vi "メイン.vi"() -> (2 "測定周期/ms":dbl, 3 "値転記用配列":T2[](array[typedef]))   [LabVIEW 2021] (continued)
                      n5618 = global write "測定値MAXMIN_G.vi" "測定値MAX/MINグローバル"(w7929) -> ()
                    }
                  }
                }
                frame 5 {
                  n5619 = local read "測定新値\nリセット用 6"() -> (w7930:bool)
                  n5620 = local read "測定旧値 6"() -> (w7931:bool)
                  n5621 = case shown="TRUE" w7930 {
                    frame False {
                    }
                    frame True {
                      n5622 = property on="MAX/MINグローバルリセット用" class="Arr (指定)"() -> ("Value"=w7932:string[][])  [unwired: 2 in, 2 out]
                      n5623 = global write "測定値MAXMIN_G.vi" "測定値MAX/MINグローバル"(w7932) -> ()
                    }
                  }
                  n5624 = case shown="TRUE" w7931 {
                    frame False {
                    }
                    frame True {
                      n5625 = property on="MAX/MINグローバルリセット用" class="Arr (指定)"() -> ("Value"=w7933:string[][])  [unwired: 2 in, 2 out]
                      n5626 = global write "測定値MAXMIN_G.vi" "測定値MAX/MINグローバル"(w7933) -> ()
                    }
                  }
                }
                frame 7 {
                  n5627 = local read "測定新値\nリセット用 8"() -> (w7934:bool)
                  n5628 = local read "測定旧値 8"() -> (w7935:bool)
                  n5629 = case shown="TRUE" w7934 {
                    frame False {
                    }
                    frame True {
                      n5630 = property on="MAX/MINグローバルリセット用" class="Arr (指定)"() -> ("Value"=w7936:string[][])  [unwired: 2 in, 2 out]
                      n5631 = global write "測定値MAXMIN_G.vi" "測定値MAX/MINグローバル"(w7936) -> ()
                    }
                  }
                  n5632 = case shown="TRUE" w7935 {
                    frame False {
                    }
                    frame True {
                      n5633 = property on="MAX/MINグローバルリセット用" class="Arr (指定)"() -> ("Value"=w7937:string[][])  [unwired: 2 in, 2 out]
                      n5634 = global write "測定値MAXMIN_G.vi" "測定値MAX/MINグローバル"(w7937) -> ()
                    }
                  }
                }
                frame 8 {
                  n5635 = local read "測定新値\nリセット用 9"() -> (w7938:bool)
                  n5636 = local read "測定旧値 9"() -> (w7939:bool)
                  n5637 = case shown="TRUE" w7938 {
                    frame False {
                    }
                    frame True {
                      n5638 = property on="MAX/MINグローバルリセット用" class="Arr (指定)"() -> ("Value"=w7940:string[][])  [unwired: 2 in, 2 out]
                      n5639 = global write "測定値MAXMIN_G.vi" "測定値MAX/MINグローバル"(w7940) -> ()
                    }
                  }
                  n5640 = case shown="TRUE" w7939 {
                    frame False {
                    }
                    frame True {
                      n5641 = property on="MAX/MINグローバルリセット用" class="Arr (指定)"() -> ("Value"=w7941:string[][])  [unwired: 2 in, 2 out]
                      n5642 = global write "測定値MAXMIN_G.vi" "測定値MAX/MINグローバル"(w7941) -> ()
                    }
                  }
                }
                frame 9 {
                  n5643 = local read "測定新値\nリセット用 10"() -> (w7942:bool)
                  n5644 = local read "測定旧値 10"() -> (w7943:bool)
                  n5645 = case shown="TRUE" w7942 {
                    frame False {
                    }
                    frame True {
                      n5646 = property on="MAX/MINグローバルリセット用" class="Arr (指定)"() -> ("Value"=w7944:string[][])  [unwired: 2 in, 2 out]
                      n5647 = global write "測定値MAXMIN_G.vi" "測定値MAX/MINグローバル"(w7944) -> ()
                    }
                  }
                  n5648 = case shown="TRUE" w7943 {
                    frame False {
                    }
                    frame True {
                      n5649 = property on="MAX/MINグローバルリセット用" class="Arr (指定)"() -> ("Value"=w7945:string[][])  [unwired: 2 in, 2 out]
                      n5650 = global write "測定値MAXMIN_G.vi" "測定値MAX/MINグローバル"(w7945) -> ()
                    }
                  }
                }
                frame 10 {
                  n5651 = local read "測定新値\nリセット用 11"() -> (w7946:bool)
                  n5652 = local read "測定旧値 11"() -> (w7947:bool)
                  n5653 = case shown="TRUE" w7946 {
                    frame False {
                    }
                    frame True {
                      n5654 = property on="MAX/MINグローバルリセット用" class="Arr (指定)"() -> ("Value"=w7948:string[][])  [unwired: 2 in, 2 out]
                      n5655 = global write "測定値MAXMIN_G.vi" "測定値MAX/MINグローバル"(w7948) -> ()
                    }
                  }
                  n5656 = case shown="TRUE" w7947 {
                    frame False {
                    }
                    frame True {
                      n5657 = property on="MAX/MINグローバルリセット用" class="Arr (指定)"() -> ("Value"=w7949:string[][])  [unwired: 2 in, 2 out]
                      n5658 = global write "測定値MAXMIN_G.vi" "測定値MAX/MINグローバル"(w7949) -> ()
                    }
                  }
                }
                frame 11 {
                  n5659 = local read "測定新値\nリセット用 12"() -> (w7950:bool)
                  n5660 = local read "測定旧値 12"() -> (w7951:bool)
                  n5661 = case shown="TRUE" w7950 {
                    frame False {
                    }
                    frame True {
                      n5662 = property on="MAX/MINグローバルリセット用" class="Arr (指定)"() -> ("Value"=w7952:string[][])  [unwired: 2 in, 2 out]
                      n5663 = global write "測定値MAXMIN_G.vi" "測定値MAX/MINグローバル"(w7952) -> ()
                    }
                  }
                  n5664 = case shown="TRUE" w7951 {
                    frame False {
                    }
                    frame True {
                      n5665 = property on="MAX/MINグローバルリセット用" class="Arr (指定)"() -> ("Value"=w7953:string[][])  [unwired: 2 in, 2 out]
                      n5666 = global write "測定値MAXMIN_G.vi" "測定値MAX/MINグローバル"(w7953) -> ()
                    }
                  }
                }
              }
            }
          }
          frame #1 {
            w7954 = FALSE
            # "②測定新規リセット用、測定旧値のリセット"
            n5667 = global write "測定キャンセルボタン.vi" "グローバル_測定キャンセルボタン"(w7954) -> ()
            n5668 = local write "G_メイン測定キャンセルボタン"(w7954) -> ()
            n5669 = for {
              N: w7955 -> [_]
              tunnel: w7954 -> [w7959]
              i -> [w7960]
              n5670 = case shown="11" w7960 {
                tunnel: w7959 -> [w7961 w7962 w7963 w7964 w7965 w7966 w7967 w7968 w7969 w7970 w7971 w7972]
                frame 0, Default {
                  n5671 = local write "測定新値\nリセット用 1"(w7961) -> ()
                  n5672 = local write "測定旧値 1"(w7961) -> ()
                }
                frame 1 {
                  n5673 = local write "測定新値\nリセット用 2"(w7962) -> ()
                  n5674 = local write "測定旧値 2"(w7962) -> ()
                }
                frame 2 {
                  n5675 = local write "測定新値\nリセット用 3"(w7963) -> ()
                  n5676 = local write "測定旧値 3"(w7963) -> ()
                }
                frame 3 {
                  n5677 = local write "測定新値\nリセット用 4"(w7964) -> ()
                  n5678 = local write "測定旧値 4"(w7964) -> ()
                }
                frame 4 {
                  n5679 = local write "測定新値\nリセット用 5"(w7965) -> ()
                  n5680 = local write "測定旧値 5"(w7965) -> ()
                }
                frame 5 {
                  n5681 = local write "測定新値\nリセット用 6"(w7966) -> ()
                  n5682 = local write "測定旧値 6"(w7966) -> ()
                }
                frame 6 {
                  n5683 = local write "測定新値\nリセット用 7"(w7967) -> ()
                  n5684 = local write "測定旧値 7"(w7967) -> ()
                }
                frame 7 {
                  n5685 = local write "測定新値\nリセット用 8"(w7968) -> ()
                  n5686 = local write "測定旧値 8"(w7968) -> ()
                }
                frame 8 {
                  n5687 = local write "測定新値\nリセット用 9"(w7969) -> ()
                  n5688 = local write "測定旧値 9"(w7969) -> ()
                }
                frame 9 {
                  n5689 = local write "測定新値\nリセット用 10"(w7970) -> ()
                  n5690 = local write "測定旧値 10"(w7970) -> ()
                }
                frame 10 {
                  n5691 = local write "測定新値\nリセット用 11"(w7971) -> ()
                  n5692 = local write "測定旧値 11"(w7971) -> ()
                }
                frame 11 {
                  n5693 = local write "測定新値\nリセット用 12"(w7972) -> ()
                  n5694 = local write "測定旧値 12"(w7972) -> ()
                }
              }
            }
          }
          frame #2 {
            # "⑦キュー"
            # "④グローバル_測定キャンセルボタンを\n対象測定新値がFalseならTrueにする"
            n5695 = case shown="TRUE" w7975 {
              tunnel: [_ w7985] -> w7979
              tunnel: w7978 -> [_ w7984]
              tunnel: [_ w7983] -> w7977
              tunnel: w7976 -> [_ w7982]
              tunnel: [w7980 w7981] -> w7974
              tunnel: [w7980 w7981] -> w7973
              frame False {
                w7980 = TRUE
              }
              frame True {
                w7981 = TRUE
                n5696 = Enqueue Element(queue=w7984, element="測定7", error in (no error)=w7982) -> (queue out=w7985:refnum<queue>, error out=w7983:errorcluster)  [unwired: 1 in, 1 out]
              }
            }
            n5697 = local write "G_メイン測定キャンセルボタン"(w7974) -> ()
            n5698 = global write "測定キャンセルボタン.vi" "グローバル_測定キャンセルボタン"(w7973) -> ()
          }
        }
        n5699 = for {
          N: 12 -> [_]
          tunnel: w7877 -> [w7891]
          i -> [w7892]
          n5700 = case shown="11" w7892 {
            tunnel: w7891 -> [w7893 w7894 w7895 w7896 w7897 w7898 w7899 w7900 w7901 w7902 w7903 w7904]
            frame 0, Default {
              n5701 = property on="メイン測定ボタン_単発 1" class="Bool (指定)"("DisabledEnum"=w7893) -> ()  [unwired: 2 in, 2 out]
              n5702 = property on="メイン測定ボタン_連続 1" class="Bool (指定)"("DisabledEnum"=w7893) -> ()  [unwired: 2 in, 2 out]
            }
            frame 1 {
              n5703 = property on="メイン測定ボタン_単発 2" class="Bool (指定)"("DisabledEnum"=w7894) -> ()  [unwired: 2 in, 2 out]
              n5704 = property on="メイン測定ボタン_連続 2" class="Bool (指定)"("DisabledEnum"=w7894) -> ()  [unwired: 2 in, 2 out]
            }
            frame 2 {
              n5705 = property on="メイン測定ボタン_単発 3" class="Bool (指定)"("DisabledEnum"=w7895) -> ()  [unwired: 2 in, 2 out]
              n5706 = property on="メイン測定ボタン_連続 3" class="Bool (指定)"("DisabledEnum"=w7895) -> ()  [unwired: 2 in, 2 out]
            }
            frame 3 {
              n5707 = property on="メイン測定ボタン_単発 4" class="Bool (指定)"("DisabledEnum"=w7896) -> ()  [unwired: 2 in, 2 out]
              n5708 = property on="メイン測定ボタン_連続 4" class="Bool (指定)"("DisabledEnum"=w7896) -> ()  [unwired: 2 in, 2 out]
            }
            frame 4 {
              n5709 = property on="メイン測定ボタン_単発 5" class="Bool (指定)"("DisabledEnum"=w7897) -> ()  [unwired: 2 in, 2 out]
              n5710 = property on="メイン測定ボタン_連続 5" class="Bool (指定)"("DisabledEnum"=w7897) -> ()  [unwired: 2 in, 2 out]
            }
            frame 5 {
              n5711 = property on="メイン測定ボタン_連続 6" class="Bool (指定)"("DisabledEnum"=w7898) -> ()  [unwired: 2 in, 2 out]
              n5712 = property on="メイン測定ボタン_単発 6" class="Bool (指定)"("DisabledEnum"=w7898) -> ()  [unwired: 2 in, 2 out]
            }
            frame 6 {
              n5713 = property on="メイン測定ボタン_連続 7" class="Bool (指定)"("DisabledEnum"=w7899) -> ()  [unwired: 2 in, 2 out]
              n5714 = property on="メイン測定ボタン_単発 7" class="Bool (指定)"("DisabledEnum"=w7899) -> ()  [unwired: 2 in, 2 out]
            }
            frame 7 {
              n5715 = property on="メイン測定ボタン_単発 8" class="Bool (指定)"("DisabledEnum"=w7900) -> ()  [unwired: 2 in, 2 out]
              n5716 = property on="メイン測定ボタン_連続 8" class="Bool (指定)"("DisabledEnum"=w7900) -> ()  [unwired: 2 in, 2 out]
            }
            frame 8 {
              n5717 = property on="メイン測定ボタン_単発 9" class="Bool (指定)"("DisabledEnum"=w7901) -> ()  [unwired: 2 in, 2 out]
              n5718 = property on="メイン測定ボタン_連続 9" class="Bool (指定)"("DisabledEnum"=w7901) -> ()  [unwired: 2 in, 2 out]
            }
            frame 9 {
              n5719 = property on="メイン測定ボタン_単発 10" class="Bool (指定)"("DisabledEnum"=w7902) -> ()  [unwired: 2 in, 2 out]
              n5720 = property on="メイン測定ボタン_連続 10" class="Bool (指定)"("DisabledEnum"=w7902) -> ()  [unwired: 2 in, 2 out]
            }
            frame 10 {
              n5721 = property on="メイン測定ボタン_単発 11" class="Bool (指定)"("DisabledEnum"=w7903) -> ()  [unwired: 2 in, 2 out]
              n5722 = property on="メイン測定ボタン_連続 11" class="Bool (指定)"("DisabledEnum"=w7903) -> ()  [unwired: 2 in, 2 out]
            }
            frame 11 {
              n5723 = property on="メイン測定ボタン_連続 12" class="Bool (指定)"("DisabledEnum"=w7904) -> ()  [unwired: 2 in, 2 out]
              n5724 = property on="メイン測定ボタン_単発 12" class="Bool (指定)"("DisabledEnum"=w7904) -> ()  [unwired: 2 in, 2 out]
            }
          }
        }
        n5725 = property on="TOPページへ" class="Bool"("DisabledEnum"=w7877) -> ()  [unwired: 2 in, 2 out]
        n5726 = property on="保存して終了" class="Bool"("DisabledEnum"=w7877) -> ()  [unwired: 2 in, 2 out]
        n5727 = property on="保存せずに" class="Bool"("DisabledEnum"=w7877) -> ()  [unwired: 2 in, 2 out]
      }
      event Value Change {
        w7988 = T8."Disabled" ("無効")
        # "⑤"
        # "※複製時\n①このボタンで操作する以外の\n測定旧値\n測定新値\nを複製して作る\n②ある分だけの\n測定旧値\nを複製して作る\n③ある分だけの\n測定旧値\nを複製して作る\n④はそのまま\n⑤測定新値の\nボタンが複製されているか確認\n⑥Ⅰ.初期設定の\n測定新値_リセットの初期化\nを必ず作る事\n⑦キュー"
        # "単発測定ボタンを押した時、G_メインとグローバルのキャンセルボタンがFalseになり、連続測定が可能な状態になる。\n500ミリ秒後G_メインとグローバルのキャンセルボタンがTrueになり、連続測定が止まる"
        n5728 = event-data() -> ("NewVal"=w7997:T7)  [unwired: 1 in, 2 out]
        "測定新値 8" <- w7997
        n5729 = local read "書込周期/ms"() -> (w7987:dbl)
        n5730 = Wait (ms)(milliseconds to wait=w7987) -> ()  [unwired: 1 out]
        n5731 = flat-sequence {
          tunnel: w7997 -> [w8017]
          tunnel: w7998 -> [w8018]
          tunnel: w8000 -> [w8019]
          tunnel: [w8019] -> w7993
          tunnel: [w8018] -> w7992
          tunnel: [w8017] -> w7991
          tunnel: [w8016] -> w7990
          tunnel: [w8069] -> w7996
          tunnel: [w8068] -> w7995
          tunnel: [w8067] -> w7994
          tunnel: w7990 -> [w8066]
          tunnel: w7991 -> [w8067]
          tunnel: w7992 -> [w8068]
          tunnel: w7993 -> [w8069]
          tunnel: [w8090] -> w8001
          tunnel: [w8088] -> w7999
          tunnel: w7996 -> [w8089]
          tunnel: w7995 -> [w8087]
          tunnel: w7994 -> [w8086]
          frame #0 {
            w8016 = 32
            # "測定旧値・新値～32までTrueだったらMAX/MINグローバルリセット"
            # "①"
            n5732 = for {
              N: w8016 -> [_]
              i -> [w8020]
              n5733 = case shown="11" w8020 {
                frame 0, Default {
                  n5734 = local read "測定新値\nリセット用 1"() -> (w8021:bool)
                  n5735 = local read "測定旧値 1"() -> (w8022:bool)
                  n5736 = case shown="TRUE" w8021 {
                    frame False {
                    }
                    frame True {
                      n5737 = property on="MAX/MINグローバルリセット用" class="Arr (指定)"() -> ("Value"=w8023:string[][])  [unwired: 2 in, 2 out]
                      n5738 = global write "測定値MAXMIN_G.vi" "測定値MAX/MINグローバル"(w8023) -> ()
                    }
                  }
                  n5739 = case shown="TRUE" w8022 {
                    frame False {
                    }
                    frame True {
                      n5740 = property on="MAX/MINグローバルリセット用" class="Arr (指定)"() -> ("Value"=w8024:string[][])  [unwired: 2 in, 2 out]
                      n5741 = global write "測定値MAXMIN_G.vi" "測定値MAX/MINグローバル"(w8024) -> ()
                    }
                  }
                }
                frame 1 {
                  n5742 = local read "測定新値\nリセット用 2"() -> (w8025:bool)
                  n5743 = local read "測定旧値 2"() -> (w8026:bool)
                  n5744 = case shown="TRUE" w8025 {
                    frame False {
                    }
                    frame True {
                      n5745 = property on="MAX/MINグローバルリセット用" class="Arr (指定)"() -> ("Value"=w8027:string[][])  [unwired: 2 in, 2 out]
                      n5746 = global write "測定値MAXMIN_G.vi" "測定値MAX/MINグローバル"(w8027) -> ()
                    }
                  }
                  n5747 = case shown="TRUE" w8026 {
                    frame False {
                    }
                    frame True {
                      n5748 = property on="MAX/MINグローバルリセット用" class="Arr (指定)"() -> ("Value"=w8028:string[][])  [unwired: 2 in, 2 out]
                      n5749 = global write "測定値MAXMIN_G.vi" "測定値MAX/MINグローバル"(w8028) -> ()
                    }
                  }
                }
                frame 2 {
                  n5750 = local read "測定新値\nリセット用 3"() -> (w8029:bool)
                  n5751 = local read "測定旧値 3"() -> (w8030:bool)
                  n5752 = case shown="TRUE" w8029 {
                    frame False {
                    }
                    frame True {
                      n5753 = property on="MAX/MINグローバルリセット用" class="Arr (指定)"() -> ("Value"=w8031:string[][])  [unwired: 2 in, 2 out]
                      n5754 = global write "測定値MAXMIN_G.vi" "測定値MAX/MINグローバル"(w8031) -> ()
                    }
                  }
                  n5755 = case shown="TRUE" w8030 {
                    frame False {
                    }
                    frame True {
                      n5756 = property on="MAX/MINグローバルリセット用" class="Arr (指定)"() -> ("Value"=w8032:string[][])  [unwired: 2 in, 2 out]
                      n5757 = global write "測定値MAXMIN_G.vi" "測定値MAX/MINグローバル"(w8032) -> ()
                    }
                  }
                }
                frame 3 {
                  n5758 = local read "測定新値\nリセット用 4"() -> (w8033:bool)
                  n5759 = local read "測定旧値 4"() -> (w8034:bool)
                  n5760 = case shown="TRUE" w8033 {
                    frame False {
                    }
                    frame True {
                      n5761 = property on="MAX/MINグローバルリセット用" class="Arr (指定)"() -> ("Value"=w8035:string[][])  [unwired: 2 in, 2 out]
                      n5762 = global write "測定値MAXMIN_G.vi" "測定値MAX/MINグローバル"(w8035) -> ()
                    }
                  }
                  n5763 = case shown="TRUE" w8034 {
                    frame False {
                    }
                    frame True {
                      n5764 = property on="MAX/MINグローバルリセット用" class="Arr (指定)"() -> ("Value"=w8036:string[][])  [unwired: 2 in, 2 out]
                      n5765 = global write "測定値MAXMIN_G.vi" "測定値MAX/MINグローバル"(w8036) -> ()
                    }
                  }
                }
                frame 4 {
                  n5766 = local read "測定新値\nリセット用 5"() -> (w8037:bool)
                  n5767 = local read "測定旧値 5"() -> (w8038:bool)
                  n5768 = case shown="TRUE" w8037 {
                    frame False {
                    }
                    frame True {
                      n5769 = property on="MAX/MINグローバルリセット用" class="Arr (指定)"() -> ("Value"=w8039:string[][])  [unwired: 2 in, 2 out]
                      n5770 = global write "測定値MAXMIN_G.vi" "測定値MAX/MINグローバル"(w8039) -> ()
                    }
                  }
                  n5771 = case shown="TRUE" w8038 {
                    frame False {
                    }
                    frame True {
                      n5772 = property on="MAX/MINグローバルリセット用" class="Arr (指定)"() -> ("Value"=w8040:string[][])  [unwired: 2 in, 2 out]
                      n5773 = global write "測定値MAXMIN_G.vi" "測定値MAX/MINグローバル"(w8040) -> ()
                    }
                  }
                }
                frame 5 {
                  n5774 = local read "測定新値\nリセット用 6"() -> (w8041:bool)
                  n5775 = local read "測定旧値 6"() -> (w8042:bool)
                  n5776 = case shown="TRUE" w8041 {
                    frame False {
                    }
                    frame True {
                      n5777 = property on="MAX/MINグローバルリセット用" class="Arr (指定)"() -> ("Value"=w8043:string[][])  [unwired: 2 in, 2 out]
                      n5778 = global write "測定値MAXMIN_G.vi" "測定値MAX/MINグローバル"(w8043) -> ()
                    }
                  }
                  n5779 = case shown="TRUE" w8042 {
                    frame False {
                    }
                    frame True {
                      n5780 = property on="MAX/MINグローバルリセット用" class="Arr (指定)"() -> ("Value"=w8044:string[][])  [unwired: 2 in, 2 out]
                      n5781 = global write "測定値MAXMIN_G.vi" "測定値MAX/MINグローバル"(w8044) -> ()
                    }
                  }
                }
                frame 6 {
                  n5782 = local read "測定新値\nリセット用 7"() -> (w8045:bool)
                  n5783 = local read "測定旧値 7"() -> (w8046:bool)
                  n5784 = case shown="TRUE" w8045 {
                    frame False {
                    }
                    frame True {
                      n5785 = property on="MAX/MINグローバルリセット用" class="Arr (指定)"() -> ("Value"=w8047:string[][])  [unwired: 2 in, 2 out]
                      n5786 = global write "測定値MAXMIN_G.vi" "測定値MAX/MINグローバル"(w8047) -> ()
                    }
                  }
                  n5787 = case shown="TRUE" w8046 {
                    frame False {
                    }
                    frame True {
                      n5788 = property on="MAX/MINグローバルリセット用" class="Arr (指定)"() -> ("Value"=w8048:string[][])  [unwired: 2 in, 2 out]
                      n5789 = global write "測定値MAXMIN_G.vi" "測定値MAX/MINグローバル"(w8048) -> ()
                    }
                  }
                }
                frame 8 {
                  n5790 = local read "測定新値\nリセット用 9"() -> (w8049:bool)
                  n5791 = local read "測定旧値 9"() -> (w8050:bool)
                  n5792 = case shown="TRUE" w8049 {
                    frame False {
                    }
                    frame True {
                      n5793 = property on="MAX/MINグローバルリセット用" class="Arr (指定)"() -> ("Value"=w8051:string[][])  [unwired: 2 in, 2 out]
                      n5794 = global write "測定値MAXMIN_G.vi" "測定値MAX/MINグローバル"(w8051) -> ()
                    }
                  }
                  n5795 = case shown="TRUE" w8050 {
                    frame False {
                    }
                    frame True {
                      n5796 = property on="MAX/MINグローバルリセット用" class="Arr (指定)"() -> ("Value"=w8052:string[][])  [unwired: 2 in, 2 out]
                      n5797 = global write "測定値MAXMIN_G.vi" "測定値MAX/MINグローバル"(w8052) -> ()
                    }
                  }
                }
                frame 9 {
                  n5798 = local read "測定新値\nリセット用 10"() -> (w8053:bool)
                  n5799 = local read "測定旧値 10"() -> (w8054:bool)
                  n5800 = case shown="TRUE" w8053 {
                    frame False {
                    }
                    frame True {
                      n5801 = property on="MAX/MINグローバルリセット用" class="Arr (指定)"() -> ("Value"=w8055:string[][])  [unwired: 2 in, 2 out]
                      n5802 = global write "測定値MAXMIN_G.vi" "測定値MAX/MINグローバル"(w8055) -> ()
                    }
                  }
                  n5803 = case shown="TRUE" w8054 {
                    frame False {
                    }
                    frame True {
                      n5804 = property on="MAX/MINグローバルリセット用" class="Arr (指定)"() -> ("Value"=w8056:string[][])  [unwired: 2 in, 2 out]
                      n5805 = global write "測定値MAXMIN_G.vi" "測定値MAX/MINグローバル"(w8056) -> ()
                    }
                  }
                }
                frame 10 {
                  n5806 = local read "測定新値\nリセット用 11"() -> (w8057:bool)
                  n5807 = local read "測定旧値 11"() -> (w8058:bool)
                  n5808 = case shown="TRUE" w8057 {
                    frame False {
                    }
                    frame True {
                      n5809 = property on="MAX/MINグローバルリセット用" class="Arr (指定)"() -> ("Value"=w8059:string[][])  [unwired: 2 in, 2 out]
                      n5810 = global write "測定値MAXMIN_G.vi" "測定値MAX/MINグローバル"(w8059) -> ()
                    }
                  }
                  n5811 = case shown="TRUE" w8058 {
                    frame False {
                    }
                    frame True {
                      n5812 = property on="MAX/MINグローバルリセット用" class="Arr (指定)"() -> ("Value"=w8060:string[][])  [unwired: 2 in, 2 out]
                      n5813 = global write "測定値MAXMIN_G.vi" "測定値MAX/MINグローバル"(w8060) -> ()
                    }
                  }
                }
                frame 11 {
                  n5814 = local read "測定新値\nリセット用 12"() -> (w8061:bool)
                  n5815 = local read "測定旧値 12"() -> (w8062:bool)
                  n5816 = case shown="TRUE" w8061 {
                    frame False {
                    }
                    frame True {
                      n5817 = property on="MAX/MINグローバルリセット用" class="Arr (指定)"() -> ("Value"=w8063:string[][])  [unwired: 2 in, 2 out]
                      n5818 = global write "測定値MAXMIN_G.vi" "測定値MAX/MINグローバル"(w8063) -> ()
                    }
                  }
                  n5819 = case shown="TRUE" w8062 {
                    frame False {
                    }
                    frame True {
                      n5820 = property on="MAX/MINグローバルリセット用" class="Arr (指定)"() -> ("Value"=w8064:string[][])  [unwired: 2 in, 2 out]
                      n5821 = global write "測定値MAXMIN_G.vi" "測定値MAX/MINグローバル"(w8064) -> ()
                    }
                  }
                }
              }
            }
          }
          frame #1 {
            w8065 = FALSE
            # "②測定新規リセット用、測定旧値のリセット"
            n5822 = global write "測定キャンセルボタン.vi" "グローバル_測定キャンセルボタン"(w8065) -> ()
            n5823 = local write "G_メイン測定キャンセルボタン"(w8065) -> ()
            n5824 = for {
              N: w8066 -> [_]
              tunnel: w8065 -> [w8070]
              i -> [w8071]
              n5825 = case shown="11" w8071 {
                tunnel: w8070 -> [w8072 w8073 w8074 w8075 w8076 w8077 w8078 w8079 w8080 w8081 w8082 w8083]
                frame 0, Default {
                  n5826 = local write "測定新値\nリセット用 1"(w8072) -> ()
                  n5827 = local write "測定旧値 1"(w8072) -> ()
                }
                frame 1 {
                  n5828 = local write "測定新値\nリセット用 2"(w8073) -> ()
                  n5829 = local write "測定旧値 2"(w8073) -> ()
                }
                frame 2 {
                  n5830 = local write "測定新値\nリセット用 3"(w8074) -> ()
                  n5831 = local write "測定旧値 3"(w8074) -> ()
                }
                frame 3 {
                  n5832 = local write "測定新値\nリセット用 4"(w8075) -> ()
                  n5833 = local write "測定旧値 4"(w8075) -> ()
                }
                frame 4 {
                  n5834 = local write "測定新値\nリセット用 5"(w8076) -> ()
                  n5835 = local write "測定旧値 5"(w8076) -> ()
                }
                frame 5 {
                  n5836 = local write "測定新値\nリセット用 6"(w8077) -> ()
                  n5837 = local write "測定旧値 6"(w8077) -> ()
                }
                frame 6 {
                  n5838 = local write "測定新値\nリセット用 7"(w8078) -> ()
                  n5839 = local write "測定旧値 7"(w8078) -> ()
                }
                frame 7 {
                  n5840 = local write "測定新値\nリセット用 8"(w8079) -> ()
                  n5841 = local write "測定旧値 8"(w8079) -> ()
                }
                frame 8 {
                  n5842 = local write "測定新値\nリセット用 9"(w8080) -> ()
                  n5843 = local write "測定旧値 9"(w8080) -> ()
                }
                frame 9 {
                  n5844 = local write "測定新値\nリセット用 10"(w8081) -> ()
                  n5845 = local write "測定旧値 10"(w8081) -> ()
                }
                frame 10 {
                  n5846 = local write "測定新値\nリセット用 11"(w8082) -> ()
                  n5847 = local write "測定旧値 11"(w8082) -> ()
                }
                frame 11 {
                  n5848 = local write "測定新値\nリセット用 12"(w8083) -> ()
                  n5849 = local write "測定旧値 12"(w8083) -> ()
                }
              }
            }
          }
          frame #2 {
            # "⑦キュー"
            # "④グローバル_測定キャンセルボタンを\n対象測定新値がFalseならTrueにする"
            n5850 = case shown="TRUE" w8086 {
              tunnel: [_ w8096] -> w8090
              tunnel: w8089 -> [_ w8095]
              tunnel: [_ w8094] -> w8088
              tunnel: w8087 -> [_ w8093]
              tunnel: [w8091 w8092] -> w8085
              tunnel: [w8091 w8092] -> w8084
              frame False {
                w8091 = TRUE
              }
              frame True {
                w8092 = TRUE
                n5851 = Enqueue Element(queue=w8095, element="測定8", error in (no error)=w8093) -> (queue out=w8096:refnum<queue>, error out=w8094:errorcluster)  [unwired: 1 in, 1 out]
              }
            }
            n5852 = local write "G_メイン測定キャンセルボタン"(w8085) -> ()
            n5853 = global write "測定キャンセルボタン.vi" "グローバル_測定キャンセルボタン"(w8084) -> ()
          }
        }
        n5854 = for {
          N: 12 -> [_]
          tunnel: w7988 -> [w8002]
          i -> [w8003]
          n5855 = case shown="11" w8003 {
            tunnel: w8002 -> [w8004 w8005 w8006 w8007 w8008 w8009 w8010 w8011 w8012 w8013 w8014 w8015]
            frame 0, Default {
              n5856 = property on="メイン測定ボタン_単発 1" class="Bool (指定)"("DisabledEnum"=w8004) -> ()  [unwired: 2 in, 2 out]
              n5857 = property on="メイン測定ボタン_連続 1" class="Bool (指定)"("DisabledEnum"=w8004) -> ()  [unwired: 2 in, 2 out]
            }
            frame 1 {
              n5858 = property on="メイン測定ボタン_単発 2" class="Bool (指定)"("DisabledEnum"=w8005) -> ()  [unwired: 2 in, 2 out]
              n5859 = property on="メイン測定ボタン_連続 2" class="Bool (指定)"("DisabledEnum"=w8005) -> ()  [unwired: 2 in, 2 out]
            }
            frame 2 {
              n5860 = property on="メイン測定ボタン_単発 3" class="Bool (指定)"("DisabledEnum"=w8006) -> ()  [unwired: 2 in, 2 out]
              n5861 = property on="メイン測定ボタン_連続 3" class="Bool (指定)"("DisabledEnum"=w8006) -> ()  [unwired: 2 in, 2 out]
            }
            frame 3 {
              n5862 = property on="メイン測定ボタン_単発 4" class="Bool (指定)"("DisabledEnum"=w8007) -> ()  [unwired: 2 in, 2 out]
              n5863 = property on="メイン測定ボタン_連続 4" class="Bool (指定)"("DisabledEnum"=w8007) -> ()  [unwired: 2 in, 2 out]
            }
            frame 4 {
              n5864 = property on="メイン測定ボタン_単発 5" class="Bool (指定)"("DisabledEnum"=w8008) -> ()  [unwired: 2 in, 2 out]
              n5865 = property on="メイン測定ボタン_連続 5" class="Bool (指定)"("DisabledEnum"=w8008) -> ()  [unwired: 2 in, 2 out]
            }
            frame 5 {
              n5866 = property on="メイン測定ボタン_連続 6" class="Bool (指定)"("DisabledEnum"=w8009) -> ()  [unwired: 2 in, 2 out]
              n5867 = property on="メイン測定ボタン_単発 6" class="Bool (指定)"("DisabledEnum"=w8009) -> ()  [unwired: 2 in, 2 out]
            }
            frame 6 {
              n5868 = property on="メイン測定ボタン_連続 7" class="Bool (指定)"("DisabledEnum"=w8010) -> ()  [unwired: 2 in, 2 out]
              n5869 = property on="メイン測定ボタン_単発 7" class="Bool (指定)"("DisabledEnum"=w8010) -> ()  [unwired: 2 in, 2 out]
            }
            frame 7 {
              n5870 = property on="メイン測定ボタン_単発 8" class="Bool (指定)"("DisabledEnum"=w8011) -> ()  [unwired: 2 in, 2 out]
              n5871 = property on="メイン測定ボタン_連続 8" class="Bool (指定)"("DisabledEnum"=w8011) -> ()  [unwired: 2 in, 2 out]
            }
            frame 8 {
              n5872 = property on="メイン測定ボタン_単発 9" class="Bool (指定)"("DisabledEnum"=w8012) -> ()  [unwired: 2 in, 2 out]
              n5873 = property on="メイン測定ボタン_連続 9" class="Bool (指定)"("DisabledEnum"=w8012) -> ()  [unwired: 2 in, 2 out]
            }
            frame 9 {
              n5874 = property on="メイン測定ボタン_単発 10" class="Bool (指定)"("DisabledEnum"=w8013) -> ()  [unwired: 2 in, 2 out]
              n5875 = property on="メイン測定ボタン_連続 10" class="Bool (指定)"("DisabledEnum"=w8013) -> ()  [unwired: 2 in, 2 out]
            }
            frame 10 {
              n5876 = property on="メイン測定ボタン_単発 11" class="Bool (指定)"("DisabledEnum"=w8014) -> ()  [unwired: 2 in, 2 out]
              n5877 = property on="メイン測定ボタン_連続 11" class="Bool (指定)"("DisabledEnum"=w8014) -> ()  [unwired: 2 in, 2 out]
            }
            frame 11 {
              n5878 = property on="メイン測定ボタン_連続 12" class="Bool (指定)"("DisabledEnum"=w8015) -> ()  [unwired: 2 in, 2 out]
              n5879 = property on="メイン測定ボタン_単発 12" class="Bool (指定)"("DisabledEnum"=w8015) -> ()  [unwired: 2 in, 2 out]
            }
          }
        }
        n5880 = property on="TOPページへ" class="Bool"("DisabledEnum"=w7988) -> ()  [unwired: 2 in, 2 out]
        n5881 = property on="保存して終了" class="Bool"("DisabledEnum"=w7988) -> ()  [unwired: 2 in, 2 out]
        n5882 = property on="保存せずに" class="Bool"("DisabledEnum"=w7988) -> ()  [unwired: 2 in, 2 out]
      }
      event Value Change {
        w8099 = T8."Disabled" ("無効")
        # "⑤"
        # "※複製時\n①このボタンで操作する以外の\n測定旧値\n測定新値\nを複製して作る\n②ある分だけの\n測定旧値\nを複製して作る\n③ある分だけの\n測定旧値\nを複製して作る\n④はそのまま\n⑤測定新値の\nボタンが複製されているか確認\n⑥Ⅰ.初期設定の\n測定新値_リセットの初期化\nを必ず作る事\n⑦キュー\n⑧ループカウント"
        # "単発測定ボタンを押した時、G_メインとグローバルのキャンセルボタンがFalseになり、連続測定が可能な状態になる。\n500ミリ秒後G_メインとグローバルのキャンセルボタンがTrueになり、連続測定が止まる"
        n5883 = event-data() -> ("NewVal"=w8108:T7)  [unwired: 1 in, 2 out]
        "測定新値 9" <- w8108
        n5884 = local read "書込周期/ms"() -> (w8098:dbl)
        n5885 = Wait (ms)(milliseconds to wait=w8098) -> ()  [unwired: 1 out]
        n5886 = flat-sequence {
          tunnel: w8108 -> [w8128]
          tunnel: w8109 -> [w8129]
          tunnel: w8111 -> [w8130]
          tunnel: [w8130] -> w8104
          tunnel: [w8129] -> w8103
          tunnel: [w8128] -> w8102
          tunnel: [w8127] -> w8101
          tunnel: [w8180] -> w8107
          tunnel: [w8179] -> w8106
          tunnel: [w8178] -> w8105
          tunnel: w8101 -> [w8177]
          tunnel: w8102 -> [w8178]
          tunnel: w8103 -> [w8179]
          tunnel: w8104 -> [w8180]
          tunnel: [w8201] -> w8112
          tunnel: [w8199] -> w8110
          tunnel: w8107 -> [w8200]
          tunnel: w8106 -> [w8198]
          tunnel: w8105 -> [w8197]
          frame #0 {
            w8127 = 32
            # "⑧"
            # "測定旧値・新値～32までTrueだったらMAX/MINグローバルリセット"
            # "①"
            n5887 = for {
              N: w8127 -> [_]
              i -> [w8131]
              n5888 = case shown="11" w8131 {
                frame 0, Default {
                  n5889 = local read "測定新値\nリセット用 1"() -> (w8132:bool)
                  n5890 = local read "測定旧値 1"() -> (w8133:bool)
                  n5891 = case shown="FALSE" w8132 {
                    frame False {
                    }
                    frame True {
                      n5892 = property on="MAX/MINグローバルリセット用" class="Arr (指定)"() -> ("Value"=w8134:string[][])  [unwired: 2 in, 2 out]
                      n5893 = global write "測定値MAXMIN_G.vi" "測定値MAX/MINグローバル"(w8134) -> ()
                    }
                  }
                  n5894 = case shown="FALSE" w8133 {
                    frame False {
                    }
                    frame True {
                      n5895 = property on="MAX/MINグローバルリセット用" class="Arr (指定)"() -> ("Value"=w8135:string[][])  [unwired: 2 in, 2 out]
                      n5896 = global write "測定値MAXMIN_G.vi" "測定値MAX/MINグローバル"(w8135) -> ()
                    }
                  }
                }
                frame 1 {
                  n5897 = local read "測定新値\nリセット用 2"() -> (w8136:bool)
                  n5898 = local read "測定旧値 2"() -> (w8137:bool)
                  n5899 = case shown="FALSE" w8136 {
                    frame False {
                    }
                    frame True {
                      n5900 = property on="MAX/MINグローバルリセット用" class="Arr (指定)"() -> ("Value"=w8138:string[][])  [unwired: 2 in, 2 out]
                      n5901 = global write "測定値MAXMIN_G.vi" "測定値MAX/MINグローバル"(w8138) -> ()
                    }
                  }
                  n5902 = case shown="FALSE" w8137 {
                    frame False {
                    }
                    frame True {
                      n5903 = property on="MAX/MINグローバルリセット用" class="Arr (指定)"() -> ("Value"=w8139:string[][])  [unwired: 2 in, 2 out]
                      n5904 = global write "測定値MAXMIN_G.vi" "測定値MAX/MINグローバル"(w8139) -> ()
                    }
                  }
                }
                frame 2 {
                  n5905 = local read "測定新値\nリセット用 3"() -> (w8140:bool)
                  n5906 = local read "測定旧値 3"() -> (w8141:bool)
                  n5907 = case shown="FALSE" w8140 {
                    frame False {
                    }
                    frame True {
                      n5908 = property on="MAX/MINグローバルリセット用" class="Arr (指定)"() -> ("Value"=w8142:string[][])  [unwired: 2 in, 2 out]
                      n5909 = global write "測定値MAXMIN_G.vi" "測定値MAX/MINグローバル"(w8142) -> ()
                    }
                  }
                  n5910 = case shown="FALSE" w8141 {
                    frame False {
                    }
                    frame True {
                      n5911 = property on="MAX/MINグローバルリセット用" class="Arr (指定)"() -> ("Value"=w8143:string[][])  [unwired: 2 in, 2 out]
                      n5912 = global write "測定値MAXMIN_G.vi" "測定値MAX/MINグローバル"(w8143) -> ()
                    }
                  }
                }
                frame 3 {
                  n5913 = local read "測定新値\nリセット用 4"() -> (w8144:bool)
                  n5914 = local read "測定旧値 4"() -> (w8145:bool)
                  n5915 = case shown="FALSE" w8144 {
                    frame False {
                    }
                    frame True {
                      n5916 = property on="MAX/MINグローバルリセット用" class="Arr (指定)"() -> ("Value"=w8146:string[][])  [unwired: 2 in, 2 out]
                      n5917 = global write "測定値MAXMIN_G.vi" "測定値MAX/MINグローバル"(w8146) -> ()
                    }
                  }
                  n5918 = case shown="FALSE" w8145 {
                    frame False {
                    }
                    frame True {
                      n5919 = property on="MAX/MINグローバルリセット用" class="Arr (指定)"() -> ("Value"=w8147:string[][])  [unwired: 2 in, 2 out]
                      n5920 = global write "測定値MAXMIN_G.vi" "測定値MAX/MINグローバル"(w8147) -> ()
                    }
                  }
                }
                frame 4 {
                  n5921 = local read "測定新値\nリセット用 5"() -> (w8148:bool)
                  n5922 = local read "測定旧値 5"() -> (w8149:bool)
                  n5923 = case shown="FALSE" w8148 {
                    frame False {
                    }
                    frame True {
                      n5924 = property on="MAX/MINグローバルリセット用" class="Arr (指定)"() -> ("Value"=w8150:string[][])  [unwired: 2 in, 2 out]
                      n5925 = global write "測定値MAXMIN_G.vi" "測定値MAX/MINグローバル"(w8150) -> ()
                    }
                  }
                  n5926 = case shown="FALSE" w8149 {
                    frame False {
                    }
                    frame True {
                      n5927 = property on="MAX/MINグローバルリセット用" class="Arr (指定)"() -> ("Value"=w8151:string[][])  [unwired: 2 in, 2 out]
                      n5928 = global write "測定値MAXMIN_G.vi" "測定値MAX/MINグローバル"(w8151) -> ()
                    }
                  }
                }
                frame 5 {
                  n5929 = local read "測定新値\nリセット用 6"() -> (w8152:bool)
                  n5930 = local read "測定旧値 6"() -> (w8153:bool)
                  n5931 = case shown="FALSE" w8152 {
                    frame False {
                    }
                    frame True {
                      n5932 = property on="MAX/MINグローバルリセット用" class="Arr (指定)"() -> ("Value"=w8154:string[][])  [unwired: 2 in, 2 out]
                      n5933 = global write "測定値MAXMIN_G.vi" "測定値MAX/MINグローバル"(w8154) -> ()
                    }
                  }
                  n5934 = case shown="FALSE" w8153 {
                    frame False {
                    }
                    frame True {
                      n5935 = property on="MAX/MINグローバルリセット用" class="Arr (指定)"() -> ("Value"=w8155:string[][])  [unwired: 2 in, 2 out]
                      n5936 = global write "測定値MAXMIN_G.vi" "測定値MAX/MINグローバル"(w8155) -> ()
                    }
                  }
                }
                frame 6 {
                  n5937 = local read "測定新値\nリセット用 7"() -> (w8156:bool)
                  n5938 = local read "測定旧値 7"() -> (w8157:bool)
                  n5939 = case shown="FALSE" w8156 {
                    frame False {
                    }
                    frame True {
                      n5940 = property on="MAX/MINグローバルリセット用" class="Arr (指定)"() -> ("Value"=w8158:string[][])  [unwired: 2 in, 2 out]
                      n5941 = global write "測定値MAXMIN_G.vi" "測定値MAX/MINグローバル"(w8158) -> ()
                    }
                  }
                  n5942 = case shown="FALSE" w8157 {
                    frame False {
                    }
                    frame True {
                      n5943 = property on="MAX/MINグローバルリセット用" class="Arr (指定)"() -> ("Value"=w8159:string[][])  [unwired: 2 in, 2 out]
                      n5944 = global write "測定値MAXMIN_G.vi" "測定値MAX/MINグローバル"(w8159) -> ()
                    }
                  }
                }
                frame 7 {
                  n5945 = local read "測定新値\nリセット用 8"() -> (w8160:bool)
                  n5946 = local read "測定旧値 8"() -> (w8161:bool)
                  n5947 = case shown="TRUE" w8160 {
                    frame False {
                    }
                    frame True {
                      n5948 = property on="MAX/MINグローバルリセット用" class="Arr (指定)"() -> ("Value"=w8162:string[][])  [unwired: 2 in, 2 out]
                      n5949 = global write "測定値MAXMIN_G.vi" "測定値MAX/MINグローバル"(w8162) -> ()
                    }
                  }
                  n5950 = case shown="TRUE" w8161 {
                    frame False {
                    }
                    frame True {
                      n5951 = property on="MAX/MINグローバルリセット用" class="Arr (指定)"() -> ("Value"=w8163:string[][])  [unwired: 2 in, 2 out]
                      n5952 = global write "測定値MAXMIN_G.vi" "測定値MAX/MINグローバル"(w8163) -> ()
                    }
                  }
                }
                frame 9 {
                  n5953 = local read "測定新値\nリセット用 10"() -> (w8164:bool)
                  n5954 = local read "測定旧値 10"() -> (w8165:bool)
                  n5955 = case shown="TRUE" w8164 {
                    frame False {
                    }
                    frame True {
                      n5956 = property on="MAX/MINグローバルリセット用" class="Arr (指定)"() -> ("Value"=w8166:string[][])  [unwired: 2 in, 2 out]
                      n5957 = global write "測定値MAXMIN_G.vi" "測定値MAX/MINグローバル"(w8166) -> ()
                    }
                  }
                  n5958 = case shown="TRUE" w8165 {
                    frame False {
                    }
                    frame True {
                      n5959 = property on="MAX/MINグローバルリセット用" class="Arr (指定)"() -> ("Value"=w8167:string[][])  [unwired: 2 in, 2 out]
                      n5960 = global write "測定値MAXMIN_G.vi" "測定値MAX/MINグローバル"(w8167) -> ()
                    }
                  }
                }
                frame 10 {
                  n5961 = local read "測定新値\nリセット用 11"() -> (w8168:bool)
                  n5962 = local read "測定旧値 11"() -> (w8169:bool)
                  n5963 = case shown="TRUE" w8168 {
                    frame False {
                    }
                    frame True {
                      n5964 = property on="MAX/MINグローバルリセット用" class="Arr (指定)"() -> ("Value"=w8170:string[][])  [unwired: 2 in, 2 out]
                      n5965 = global write "測定値MAXMIN_G.vi" "測定値MAX/MINグローバル"(w8170) -> ()
                    }
                  }
                  n5966 = case shown="TRUE" w8169 {
                    frame False {
                    }
                    frame True {
                      n5967 = property on="MAX/MINグローバルリセット用" class="Arr (指定)"() -> ("Value"=w8171:string[][])  [unwired: 2 in, 2 out]
                      n5968 = global write "測定値MAXMIN_G.vi" "測定値MAX/MINグローバル"(w8171) -> ()
                    }
                  }
                }
                frame 11 {
                  n5969 = local read "測定新値\nリセット用 12"() -> (w8172:bool)
                  n5970 = local read "測定旧値 12"() -> (w8173:bool)
                  n5971 = case shown="TRUE" w8172 {
                    frame False {
                    }
                    frame True {
                      n5972 = property on="MAX/MINグローバルリセット用" class="Arr (指定)"() -> ("Value"=w8174:string[][])  [unwired: 2 in, 2 out]
                      n5973 = global write "測定値MAXMIN_G.vi" "測定値MAX/MINグローバル"(w8174) -> ()
                    }
                  }
                  n5974 = case shown="TRUE" w8173 {
                    frame False {
                    }
                    frame True {
                      n5975 = property on="MAX/MINグローバルリセット用" class="Arr (指定)"() -> ("Value"=w8175:string[][])  [unwired: 2 in, 2 out]
                      n5976 = global write "測定値MAXMIN_G.vi" "測定値MAX/MINグローバル"(w8175) -> ()
                    }
                  }
                }
              }
            }
          }
          frame #1 {
            w8176 = FALSE
            # "②測定新規リセット用、測定旧値のリセット"
            n5977 = for {
              N: w8177 -> [_]
              tunnel: w8176 -> [w8181]
              i -> [w8182]
              n5978 = case shown="11" w8182 {
                tunnel: w8181 -> [w8183 w8184 w8185 w8186 w8187 w8188 w8189 w8190 w8191 w8192 w8193 w8194]
                frame 0, Default {
                  n5979 = local write "測定新値\nリセット用 1"(w8183) -> ()
                  n5980 = local write "測定旧値 1"(w8183) -> ()
                }
                frame 1 {
                  n5981 = local write "測定新値\nリセット用 2"(w8184) -> ()
                  n5982 = local write "測定旧値 2"(w8184) -> ()
                }
                frame 2 {
                  n5983 = local write "測定新値\nリセット用 3"(w8185) -> ()
                  n5984 = local write "測定旧値 3"(w8185) -> ()
                }
                frame 3 {
                  n5985 = local write "測定新値\nリセット用 4"(w8186) -> ()
                  n5986 = local write "測定旧値 4"(w8186) -> ()
                }
                frame 4 {
                  n5987 = local write "測定新値\nリセット用 5"(w8187) -> ()
                  n5988 = local write "測定旧値 5"(w8187) -> ()
                }
                frame 5 {
                  n5989 = local write "測定新値\nリセット用 6"(w8188) -> ()
                  n5990 = local write "測定旧値 6"(w8188) -> ()
                }
                frame 6 {
                  n5991 = local write "測定新値\nリセット用 7"(w8189) -> ()
                  n5992 = local write "測定旧値 7"(w8189) -> ()
                }
                frame 7 {
                  n5993 = local write "測定新値\nリセット用 8"(w8190) -> ()
                  n5994 = local write "測定旧値 8"(w8190) -> ()
                }
                frame 8 {
                  n5995 = local write "測定新値\nリセット用 9"(w8191) -> ()
                  n5996 = local write "測定旧値 9"(w8191) -> ()
                }
                frame 9 {
                  n5997 = local write "測定新値\nリセット用 10"(w8192) -> ()
                  n5998 = local write "測定旧値 10"(w8192) -> ()
                }
                frame 10 {
                  n5999 = local write "測定新値\nリセット用 11"(w8193) -> ()
                  n6000 = local write "測定旧値 11"(w8193) -> ()
                }
                frame 11 {
                  n6001 = local write "測定新値\nリセット用 12"(w8194) -> ()
                  n6002 = local write "測定旧値 12"(w8194) -> ()
                }
              }
            }
            n6003 = global write "測定キャンセルボタン.vi" "グローバル_測定キャンセルボタン"(w8176) -> ()
            n6004 = local write "G_メイン測定キャンセルボタン"(w8176) -> ()
          }
          frame #2 {
            # "⑦キュー"
            # "④グローバル_測定キャンセルボタンを\n対象測定新値がFalseならTrueにする"
            n6005 = case shown="TRUE" w8197 {
              tunnel: [_ w8207] -> w8201
              tunnel: w8200 -> [_ w8206]
              tunnel: [_ w8205] -> w8199
              tunnel: w8198 -> [_ w8204]
              tunnel: [w8202 w8203] -> w8196
              tunnel: [w8202 w8203] -> w8195
              frame False {
                w8202 = TRUE
              }
              frame True {
                w8203 = TRUE
                n6006 = Enqueue Element(queue=w8206, element="測定9", error in (no error)=w8204) -> (queue out=w8207:refnum<queue>, error out=w8205:errorcluster)  [unwired: 1 in, 1 out]
              }
            }
            n6007 = local write "G_メイン測定キャンセルボタン"(w8196) -> ()
            n6008 = global write "測定キャンセルボタン.vi" "グローバル_測定キャンセルボタン"(w8195) -> ()
          }
        }
        n6009 = for {
          N: 12 -> [_]
          tunnel: w8099 -> [w8113]
          i -> [w8114]
          n6010 = case shown="11" w8114 {
            tunnel: w8113 -> [w8115 w8116 w8117 w8118 w8119 w8120 w8121 w8122 w8123 w8124 w8125 w8126]
            frame 0, Default {
              n6011 = property on="メイン測定ボタン_単発 1" class="Bool (指定)"("DisabledEnum"=w8115) -> ()  [unwired: 2 in, 2 out]
              n6012 = property on="メイン測定ボタン_連続 1" class="Bool (指定)"("DisabledEnum"=w8115) -> ()  [unwired: 2 in, 2 out]
            }
            frame 1 {
              n6013 = property on="メイン測定ボタン_単発 2" class="Bool (指定)"("DisabledEnum"=w8116) -> ()  [unwired: 2 in, 2 out]
              n6014 = property on="メイン測定ボタン_連続 2" class="Bool (指定)"("DisabledEnum"=w8116) -> ()  [unwired: 2 in, 2 out]
            }
            frame 2 {
              n6015 = property on="メイン測定ボタン_単発 3" class="Bool (指定)"("DisabledEnum"=w8117) -> ()  [unwired: 2 in, 2 out]
              n6016 = property on="メイン測定ボタン_連続 3" class="Bool (指定)"("DisabledEnum"=w8117) -> ()  [unwired: 2 in, 2 out]
            }
            frame 3 {
              n6017 = property on="メイン測定ボタン_単発 4" class="Bool (指定)"("DisabledEnum"=w8118) -> ()  [unwired: 2 in, 2 out]
              n6018 = property on="メイン測定ボタン_連続 4" class="Bool (指定)"("DisabledEnum"=w8118) -> ()  [unwired: 2 in, 2 out]
            }
            frame 4 {
              n6019 = property on="メイン測定ボタン_単発 5" class="Bool (指定)"("DisabledEnum"=w8119) -> ()  [unwired: 2 in, 2 out]
              n6020 = property on="メイン測定ボタン_連続 5" class="Bool (指定)"("DisabledEnum"=w8119) -> ()  [unwired: 2 in, 2 out]
            }
            frame 5 {
              n6021 = property on="メイン測定ボタン_連続 6" class="Bool (指定)"("DisabledEnum"=w8120) -> ()  [unwired: 2 in, 2 out]
              n6022 = property on="メイン測定ボタン_単発 6" class="Bool (指定)"("DisabledEnum"=w8120) -> ()  [unwired: 2 in, 2 out]
            }
            frame 6 {
              n6023 = property on="メイン測定ボタン_連続 7" class="Bool (指定)"("DisabledEnum"=w8121) -> ()  [unwired: 2 in, 2 out]
              n6024 = property on="メイン測定ボタン_単発 7" class="Bool (指定)"("DisabledEnum"=w8121) -> ()  [unwired: 2 in, 2 out]
            }
            frame 7 {
              n6025 = property on="メイン測定ボタン_単発 8" class="Bool (指定)"("DisabledEnum"=w8122) -> ()  [unwired: 2 in, 2 out]
              n6026 = property on="メイン測定ボタン_連続 8" class="Bool (指定)"("DisabledEnum"=w8122) -> ()  [unwired: 2 in, 2 out]
            }
            frame 8 {
              n6027 = property on="メイン測定ボタン_単発 9" class="Bool (指定)"("DisabledEnum"=w8123) -> ()  [unwired: 2 in, 2 out]
              n6028 = property on="メイン測定ボタン_連続 9" class="Bool (指定)"("DisabledEnum"=w8123) -> ()  [unwired: 2 in, 2 out]
            }
            frame 9 {
              n6029 = property on="メイン測定ボタン_単発 10" class="Bool (指定)"("DisabledEnum"=w8124) -> ()  [unwired: 2 in, 2 out]
              n6030 = property on="メイン測定ボタン_連続 10" class="Bool (指定)"("DisabledEnum"=w8124) -> ()  [unwired: 2 in, 2 out]
            }
            frame 10 {
              n6031 = property on="メイン測定ボタン_単発 11" class="Bool (指定)"("DisabledEnum"=w8125) -> ()  [unwired: 2 in, 2 out]
              n6032 = property on="メイン測定ボタン_連続 11" class="Bool (指定)"("DisabledEnum"=w8125) -> ()  [unwired: 2 in, 2 out]
            }
            frame 11 {
              n6033 = property on="メイン測定ボタン_連続 12" class="Bool (指定)"("DisabledEnum"=w8126) -> ()  [unwired: 2 in, 2 out]
              n6034 = property on="メイン測定ボタン_単発 12" class="Bool (指定)"("DisabledEnum"=w8126) -> ()  [unwired: 2 in, 2 out]
            }
          }
        }
        n6035 = property on="TOPページへ" class="Bool"("DisabledEnum"=w8099) -> ()  [unwired: 2 in, 2 out]
        n6036 = property on="保存して終了" class="Bool"("DisabledEnum"=w8099) -> ()  [unwired: 2 in, 2 out]
        n6037 = property on="保存せずに" class="Bool"("DisabledEnum"=w8099) -> ()  [unwired: 2 in, 2 out]
      }
      event Value Change {
        w8210 = T8."Disabled" ("無効")
        # "⑤"
        # "※複製時\n①このボタンで操作する以外の\n測定旧値\n測定新値\nを複製して作る\n②ある分だけの\n測定旧値\nを複製して作る\n③ある分だけの\n測定旧値\nを複製して作る\n④はそのまま\n⑤測定新値の\nボタンが複製されているか確認\n⑥Ⅰ.初期設定の\n測定新値_リセットの初期化\nを必ず作る事\n⑦キュー\n⑧ループカウント"
        # "単発測定ボタンを押した時、G_メインとグローバルのキャンセルボタンがFalseになり、連続測定が可能な状態になる。\n500ミリ秒後G_メインとグローバルのキャンセルボタンがTrueになり、連続測定が止まる"
        n6038 = event-data() -> ("NewVal"=w8219:T7)  [unwired: 1 in, 2 out]
        "測定新値 10" <- w8219
        n6039 = local read "書込周期/ms"() -> (w8209:dbl)
        n6040 = Wait (ms)(milliseconds to wait=w8209) -> ()  [unwired: 1 out]
        n6041 = flat-sequence {
          tunnel: w8219 -> [w8239]
          tunnel: w8220 -> [w8240]
          tunnel: w8222 -> [w8241]
          tunnel: [w8241] -> w8215
          tunnel: [w8240] -> w8214
          tunnel: [w8239] -> w8213
          tunnel: [w8238] -> w8212
          tunnel: [w8291] -> w8218
          tunnel: [w8290] -> w8217
          tunnel: [w8289] -> w8216
          tunnel: w8212 -> [w8288]
          tunnel: w8213 -> [w8289]
          tunnel: w8214 -> [w8290]
          tunnel: w8215 -> [w8291]
          tunnel: [w8312] -> w8223
          tunnel: [w8310] -> w8221
          tunnel: w8218 -> [w8311]
          tunnel: w8217 -> [w8309]
          tunnel: w8216 -> [w8308]
          frame #0 {
            w8238 = 32
            # "測定旧値・新値～32までTrueだったらMAX/MINグローバルリセット"
            # "①"
            n6042 = for {
              N: w8238 -> [_]
              i -> [w8242]
              n6043 = case shown="11" w8242 {
                frame 0, Default {
                  n6044 = local read "測定新値\nリセット用 1"() -> (w8243:bool)
                  n6045 = local read "測定旧値 1"() -> (w8244:bool)
                  n6046 = case shown="FALSE" w8243 {
                    frame False {
                    }
                    frame True {
